vi "array.vi"() -> ()   [LabVIEW 2020]
uses:
  <vilib>/numeric/Random Number (Range) U64.vi
  <vilib>/numeric/sub_Random U32.vi
panel:
  out "Array 2":u64[][](array[numeric])
  in  "number  of row":i32
  in  "numbers of col":i32
  out "Array":u64[](array[numeric])
  in  "Array size":i32
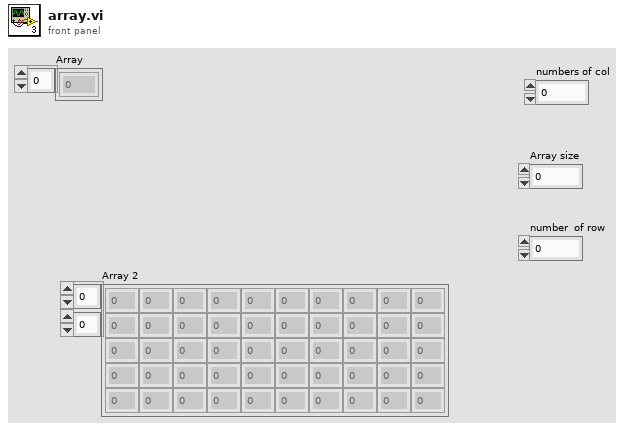
[diagram p1: front panel]
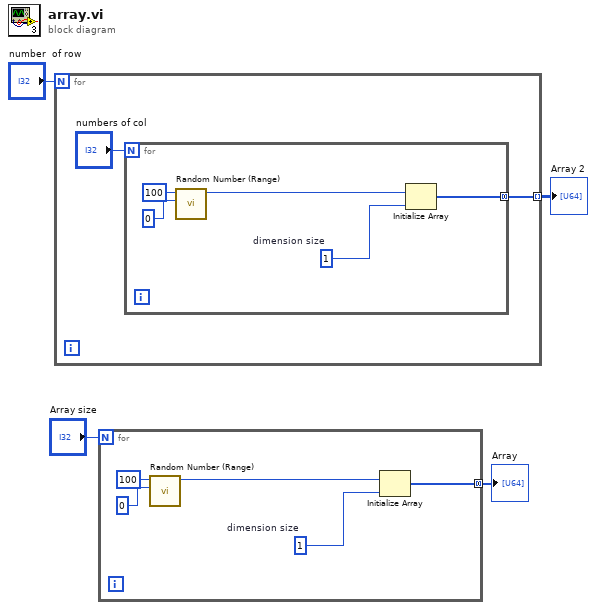
[diagram p0: block diagram]
diagram:
  n1 = for {
    N: "number  of row" -> [_]
    tunnel: [w5] -> w1 mode=indexing
    n2 = for {
      N: "numbers of col" -> [_]
      tunnel: [w7] -> w5 mode=concatenating
      w8 = 1  # dimension size
      n3 = call-poly <vilib>:"Random Number (Range).vi"("lower bound (0)"=u64 0, "upper bound (100)"=u64 100) -> ("number"=w9:u64)  [unwired: 9 in]
      n4 = Initialize Array "Initialize Array"(w9, w8) -> (w7:u64[])
    }
  }
  "Array 2" <- w1
  n5 = for {
    N: "Array size" -> [_]
    tunnel: [w12] -> w3 mode=concatenating
    w13 = 1  # dimension size
    n6 = call-poly <vilib>:"Random Number (Range).vi"("lower bound (0)"=u64 0, "upper bound (100)"=u64 100) -> ("number"=w14:u64)  [unwired: 9 in]
    n7 = Initialize Array "Initialize Array"(w14, w13) -> (w12:u64[])
  }
  "Array" <- w3
